vi "Joystick tuner.vi"(0 "Joystick Z":dbl, 2 "Loop ID":i32=3, 4 "Max":dbl=1.5, 8 "Min":dbl=0.25) -> (7 "Output":dbl)   [LabVIEW 2013]
panel:
  # "a reentrant joystick tuning utility"
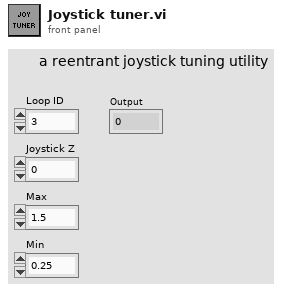
[diagram p1: front panel]
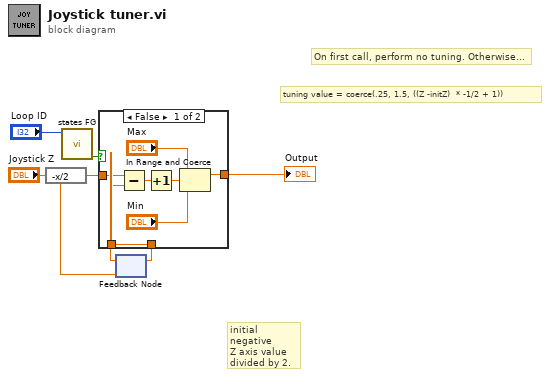
[diagram p0: block diagram]
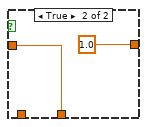
[diagram p2: hidden frame]
diagram:
  # "tuning value = coerce(.25, 1.5, ((Z -initZ)  * -1/2 + 1))"
  # "initial negative\nZ axis value\ndivided by 2."
  # "On first call, perform no tuning. Otherwise..."
  n1 = expression code="-x/2"("Joystick Z") -> (w3:dbl)
  n2 = call "states FG.vi"("Loop ID"="Loop ID") -> ("first call?"=w5:bool)  [unwired: 7 in, 3 out]
  n3 = feedback #1(w3) -> (w7:dbl)
  n4 = case shown="False" w5 {
    tunnel: w3 -> [w14 w16]
    tunnel: [w11 w16] -> w6
    tunnel: w7 -> [w11 _]
    tunnel: [w13 1.0 ("upper limit")] -> w1
    frame False {
      n5 = Subtract(x=w14, y=w11) -> (x-y=w12:dbl)
      n6 = Increment(x=w12) -> (x+1=w10:dbl)
      n7 = In Range and Coerce(upper limit="Max", x=w10, lower limit="Min") -> (coerced(x)=w13:dbl)  [unwired: 1 out]
    }
    frame True {
    }
  }
  "Output" <- w1
  n8 = feedback-in #1(w6) -> ()
